vi "Unicode (UCS32) to UTF8 Encoding.vi"(8 "error in (no error)":errorcluster, 9 "UCS 32":u32 format="%.0x") -> (0 "error out":errorcluster, 1 "[UTF-8]":u8[](array[numeric]) format="%.0x")   [LabVIEW 2011]
doc: "Converts the given Unicode in UCS 32 representation to UTF-8 Encoded Unicode string.\n\nUTF-8 is one of the Encodings to store the 21 bit Unicode numbers in a compact format.\n i.e. it stores the Unicode in one or more Byte sequences."
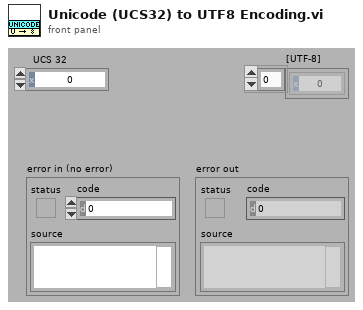
[diagram p1: front panel]
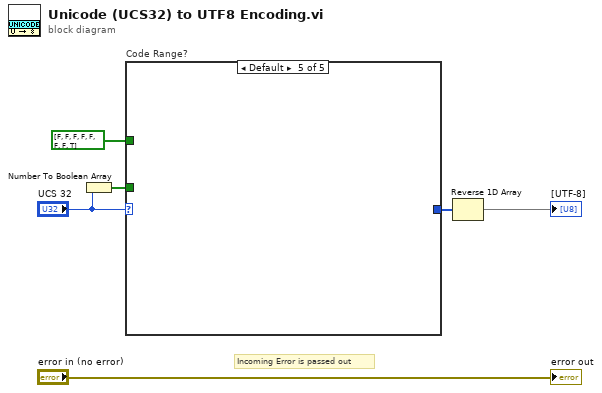
[diagram p0: block diagram]
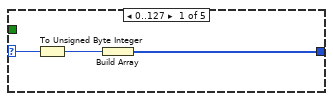
[diagram p2: hidden frame]
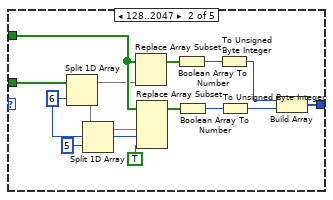
[diagram p3: hidden frame]
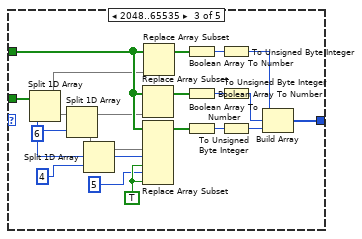
[diagram p4: hidden frame]
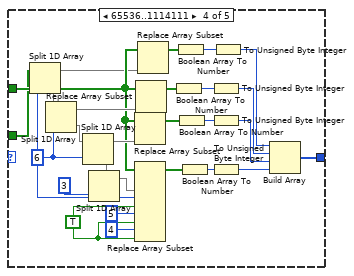
[diagram p5: hidden frame]
diagram:
  # "Incoming Error is passed out"
  n1 = Number To Boolean Array(number="UCS 32") -> (Boolean array=w6:bool[])
  n2 = case "Code Range?" shown="Default" "UCS 32" {
    selector: "UCS 32" -> [w9 _ _ _ _]
    tunnel: [w7 w15 w40 w68 _] -> w4
    tunnel: w6 -> [_ w24 w45 w53 _]
    tunnel: bool[] [FALSE, FALSE, FALSE, FALSE, FALSE, FALSE, FALSE, TRUE] -> [_ w23 w38 w55 _]
    frame 0..127 {
      n3 = To Unsigned Byte Integer(number=w9) -> (unsigned 8bit integer=w8:u8)
      n4 = Build Array(w8) -> (w7:u8[])
    }
    frame 128..2047 {
      w20 = 6 ("index")
      n5 = Split 1D Array(array=w24, index=w20) -> (first subarray=w22:bool[], second subarray=w12:bool[])
      n6 = Split 1D Array(array=w12, index=5) -> (first subarray=w11:bool[])  [unwired: 1 out]
      n7 = Replace Array Subset(array=w23, new element=w22) -> (w18:bool[])  [unwired: 1 in]
      n8 = Replace Array Subset(array=w23, new element #1=w11, new element #2=TRUE ("new element/subarray"), index #2=w20) -> (w19:bool[])  [unwired: 1 in]
      n9 = Boolean Array To Number(Boolean array=w18) -> (number=w16:u32)
      n10 = Boolean Array To Number(Boolean array=w19) -> (number=w17:u32)
      n11 = To Unsigned Byte Integer(number=w16) -> (unsigned 8bit integer=w14:u8)
      n12 = To Unsigned Byte Integer(number=w17) -> (unsigned 8bit integer=w13:u8)
      n13 = Build Array(w14, w13) -> (w15:u8[])
    }
    frame 2048..65535 {
      w35 = TRUE ("new element/subarray")
      w29 = 6 ("index")
      n14 = Split 1D Array(array=w45, index=w29) -> (first subarray=w33:bool[], second subarray=w39:bool[])
      n15 = Split 1D Array(array=w39, index=w29) -> (first subarray=w32:bool[], second subarray=w26:bool[])
      n16 = Split 1D Array(array=w26, index=4) -> (first subarray=w25:bool[])  [unwired: 1 out]
      n17 = Replace Array Subset(array=w38, new element=w32) -> (w43:bool[])  [unwired: 1 in]
      n18 = Replace Array Subset(array=w38, new element #1=w25, new element #2=w35, index #2=w29, new element #3=w35, index #3=5 ("index")) -> (w44:bool[])  [unwired: 1 in]
      n19 = Replace Array Subset(array=w38, new element=w33) -> (w36:bool[])  [unwired: 1 in]
      n20 = Boolean Array To Number(Boolean array=w36) -> (number=w37:u32)
      n21 = Boolean Array To Number(Boolean array=w43) -> (number=w41:u32)
      n22 = Boolean Array To Number(Boolean array=w44) -> (number=w42:u32)
      n23 = To Unsigned Byte Integer(number=w37) -> (unsigned 8bit integer=w30:u8)
      n24 = To Unsigned Byte Integer(number=w41) -> (unsigned 8bit integer=w31:u8)
      n25 = To Unsigned Byte Integer(number=w42) -> (unsigned 8bit integer=w34:u8)
      n26 = Build Array(w30, w31, w34) -> (w40:u8[])
    }
    frame 65536..1114111 {
      w47 = TRUE ("new element/subarray")
      w46 = 6 ("index")
      n27 = Split 1D Array(array=w53, index=w46) -> (first subarray=w51:bool[], second subarray=w52:bool[])
      n28 = Split 1D Array(array=w52, index=w46) -> (first subarray=w56:bool[], second subarray=w67:bool[])
      n29 = Split 1D Array(array=w67, index=w46) -> (first subarray=w63:bool[], second subarray=w50:bool[])
      n30 = Split 1D Array(array=w50, index=3) -> (first subarray=w49:bool[])  [unwired: 1 out]
      n31 = Replace Array Subset(array=w55, new element=w63) -> (w71:bool[])  [unwired: 1 in]
      n32 = Replace Array Subset(array=w55, new element #1=w49, new element #2=w47, index #2=w46, new element #3=w47, index #3=5 ("index"), new element #4=w47, index #4=4 ("index")) -> (w72:bool[])  [unwired: 1 in]
      n33 = Replace Array Subset(array=w55, new element=w56) -> (w65:bool[])  [unwired: 1 in]
      n34 = Replace Array Subset(array=w55, new element=w51) -> (w58:bool[])  [unwired: 1 in]
      n35 = Boolean Array To Number(Boolean array=w65) -> (number=w66:u32)
      n36 = Boolean Array To Number(Boolean array=w58) -> (number=w57:u32)
      n37 = Boolean Array To Number(Boolean array=w71) -> (number=w69:u32)
      n38 = Boolean Array To Number(Boolean array=w72) -> (number=w70:u32)
      n39 = To Unsigned Byte Integer(number=w66) -> (unsigned 8bit integer=w61:u8)
      n40 = To Unsigned Byte Integer(number=w69) -> (unsigned 8bit integer=w62:u8)
      n41 = To Unsigned Byte Integer(number=w70) -> (unsigned 8bit integer=w64:u8)
      n42 = To Unsigned Byte Integer(number=w57) -> (unsigned 8bit integer=w54:u8)
      n43 = Build Array(w54, w61, w62, w64) -> (w68:u8[])
    }
    frame Default {
    }
  }
  n44 = Reverse 1D Array(array=w4) -> (reversed array=→"[UTF-8]":u8[])
  "error out" <- "error in (no error)"
